vi "Request Subscriber by Name.vi"(8 "error in (no error)":errorcluster, 10 "Topic Name":string, 11 "Subscriber Look Up Table in":refnum<class "Subscriber Look Up Table.lvclass">) -> (0 "error out":errorcluster, 1 "Found?":bool, 2 "Subscriber":refnum<class "Message Transport Interface.lvclass">, 3 "Subscriber Look Up Table out":refnum<class "Subscriber Look Up Table.lvclass">)   [LabVIEW 2016, in "Stream Mediator.lvlib" / "Subscriber Look Up Table.lvclass"]
doc: "--\nCopyright © 2017 Composed SystemsI All rights reserved.\n\nAuthor: Jon McBee <jon.mcbee@composed.io>\n\nThis library is provided \"AS IS\" ,WITHOUT WARRANTIES OR\nCONDITIONS OF ANY KIND, either express or implied.\n\nComposed Systems -- composed.io\n\nStream 0.0.1.1\nJon McBee - Composed Systems\nCopyright (c) 2017, Composed Systems"
uses:
  <userlib>/Composed Systems/Stream/Mediator/Classes/Subscriber Look Up Table/Subscriber Look Up Table.lvclass
  C:/Program Files (x86)/National Instruments/LabVIEW 2016/user.lib/Composed Systems/Stream/Look Up Table/Look Up Table/Look Up Table.lvclass
  <userlib>/Composed Systems/Stream/Mediator/Classes/Message Transport Interface/Message Transport Interface.lvclass
  <userlib>/Composed Systems/Stream/Look Up Table/Look Up Table/Look Up Table.lvclass
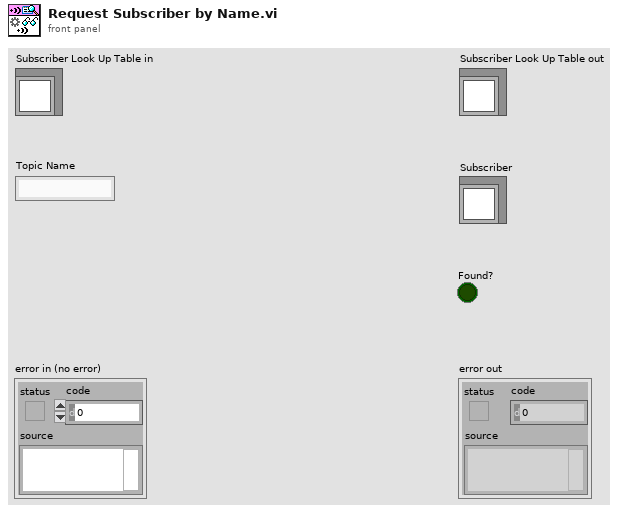
[diagram p1: front panel]
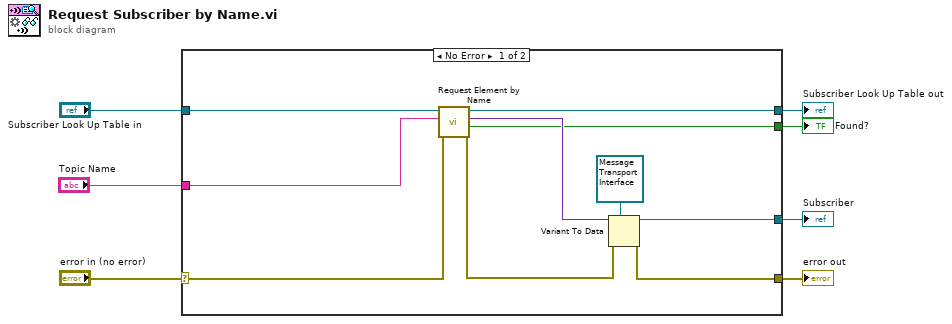
[diagram p0: block diagram]
diagram:
  n1 = case shown="No Error" "error in (no error)" {
    selector: "error in (no error)" -> [w10 w19]
    tunnel: [w17 w19] -> w6
    tunnel: [w12 w18] -> w4
    tunnel: "Subscriber Look Up Table in" -> [w14 w18]
    tunnel: "Topic Name" -> [w13 _]
    tunnel: [w15 _] -> w2
    tunnel: [w9 _] -> w1
    frame No Error {
      n2 = call <userlib>:"Request Element by Name.vi"("error in (no error)"=w10, "Name"=w13, "Look Up Table in"=w14) -> ("error out"=w8:errorcluster, "Found?"=w9:bool, "Element"=w11:variant, "Look Up Table out"=w12:refnum<class "Subscriber Look Up Table.lvclass">)  [unwired: 5 in]
      n3 = Variant To Data(error in=w8, type=refnum<class "Message Transport Interface.lvclass"> refnum ("Subscriber"), Variant=w11) -> (data=w15:refnum<class "Message Transport Interface.lvclass">, error out=w17:errorcluster)
    }
    frame Error {
    }
  }
  "error out" <- w6
  "Subscriber Look Up Table out" <- w4
  "Found?" <- w1
  "Subscriber" <- w2
